vi "Get Subscribe Data Events.vi"(11 "UserEvents in":refnum<class "User Events.lvclass">) -> (2 "Subscribe Data Events":T1, 3 "UserEvents out":refnum<class "User Events.lvclass">)   [LabVIEW 2015, in "User Events.lvclass"]
uses:
  User Events.lvclass
  Typedefs/Subscribe Data Events.ctl
  User Events.lvclass/User Events.ctl
  Typedefs/FAMT Typedefs.lvlib
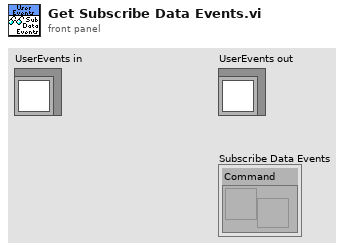
[diagram p1: front panel]
types:
  T1 = typedef "FAMT Typedefs.lvlib/Subscribe Data Events.ctl" = cluster{"Command":refnum<user-event>}
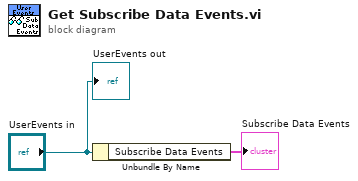
[diagram p0: block diagram]
diagram:
  n1 = Unbundle By Name("UserEvents in") -> ("Subscribe Data Events"=→"Subscribe Data Events":T1)
  "UserEvents out" <- "UserEvents in"
